vi "Write Room Cleaning.vi"(8 "error in (no error)":errorcluster, 10 "Room Cleaning":bool, 11 "Housekeeping in":refnum<class "Housekeeping.lvclass">) -> (0 "error out":errorcluster, 3 "Housekeeping out":refnum<class "Housekeeping.lvclass">)   [LabVIEW 2023, in "Room Service Types.lvlib" / "Housekeeping.lvclass"]
uses:
  Housekeeping.lvclass
  Housekeeping.lvclass/Housekeeping.ctl
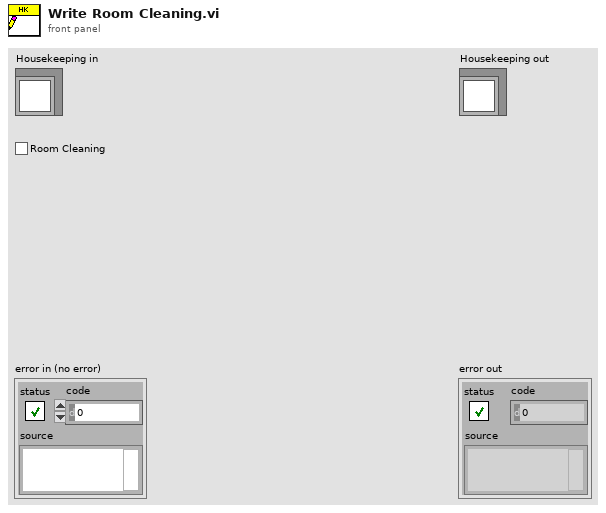
[diagram p1: front panel]
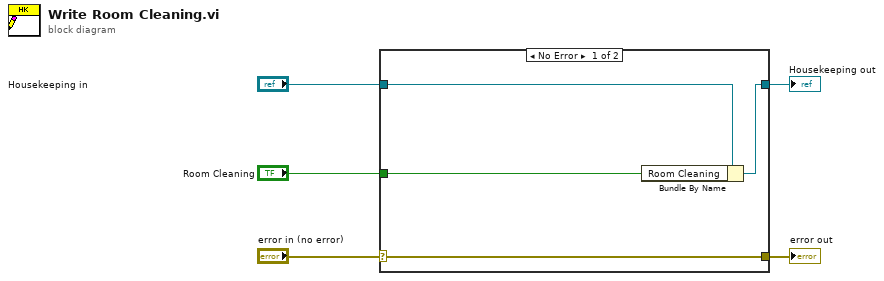
[diagram p0: block diagram]
diagram:
  n1 = case shown="No Error" "error in (no error)" {
    selector: "error in (no error)" -> [w9 w10]
    tunnel: [w9 w10] -> w4
    tunnel: [w7 w11] -> w2
    tunnel: "Housekeeping in" -> [w8 w11]
    tunnel: "Room Cleaning" -> [w6 _]
    frame No Error {
      n2 = Bundle By Name(cluster=w8, "Room Cleaning"=w6) -> (w7:refnum<class "Housekeeping.lvclass">)
    }
    frame Error {
    }
  }
  "error out" <- w4
  "Housekeeping out" <- w2
